vi "Display Error.vi"(6 "Show \"Ignore Error\" (T)":bool=TRUE, 10 "Error to Display":errorcluster, 11 "Title (\"\")":string) -> (2 "Ignore Error":bool, 3 "Exit?":bool)   [LabVIEW 2018]
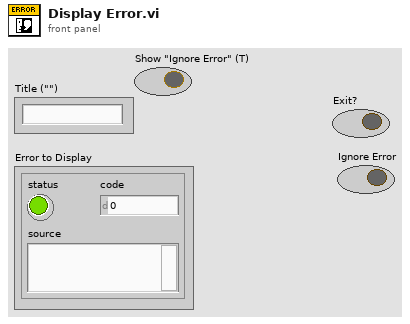
[diagram p1: front panel]
types:
  T1 = enum16{"Left Button", "Center Button", "Right Button", "Window Close"}
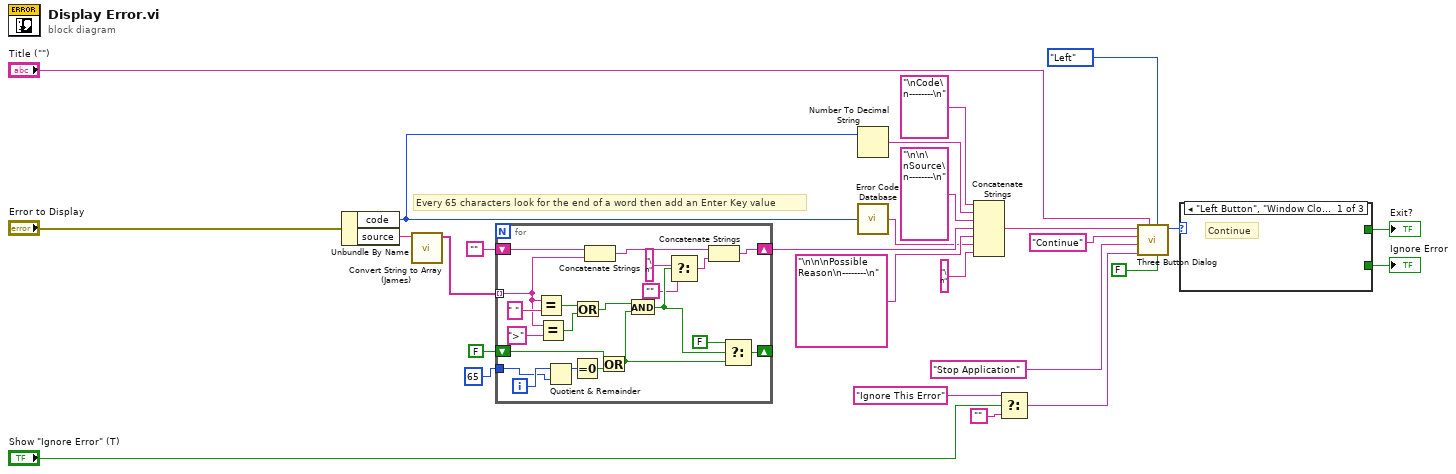
[diagram p0: block diagram]
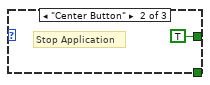
[diagram p2: hidden frame]
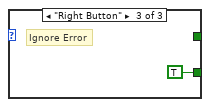
[diagram p3: hidden frame]
diagram:
  # "Every 65 characters look for the end of a word then add an Enter Key value"
  n1 = Unbundle By Name("Error to Display") -> ("code"=w17:i32, "source"=w20:string)
  n2 = call "Convert String to Array (James).vi"("String in"=w20) -> ("Array out"=w24:string[])  [unwired: 9 in, 1 out]
  n3 = for {
    tunnel: w24 -> [w42] mode=indexing
    shift-right: [w39] -> w19
    shift-left: "" -> [w47]
    tunnel: 65 ("length") -> [w28]
    shift-right: [w37] -> _
    shift-left: FALSE -> [w33]
    i -> [w29]
    n4 = Equal?(x=w42, y=" ") -> (x = y?=w43:bool)
    n5 = Equal?(x=w42, y=">") -> (x = y?=w40:bool)
    n6 = Quotient & Remainder(x=w29, y=w28) -> (x-y*floor(x/y)=w46:i32)  [unwired: 1 out]
    n7 = Equal To 0?(x=w46) -> (x = 0?=w45:bool)
    n8 = Or(x=w43, y=w40) -> (x .or. y?=w34:bool)
    n9 = Concatenate Strings(w47, w42) -> (w48:string)
    n10 = Or(x=w33, y=w45) -> (x .or. y?=w32:bool)
    n11 = And(x=w34, y=w32) -> (x .and. y?=w38:bool)
    n12 = Select(t="\n", s=w38, f="") -> (s? t:f=w35:string)
    n13 = Concatenate Strings(w48, w35) -> (w39:string)
    n14 = Select(t=FALSE, s=w38, f=w32) -> (s? t:f=w37:bool)
  }
  n15 = Number To Decimal String(number=w17) -> (decimal integer string=w27:string)  [unwired: 1 in]
  n16 = call <vilib>:"Error Code Database.vi"("Error Code"=w17) -> ("Error Text"=w16:string)
  n17 = Concatenate Strings("\nCode\n--------\n", w27, "\n\n\nSource\n--------\n", w19, "\n\n\nPossible Reason\n--------\n" ("string"), w16, "\n" ("string")) -> (w10:string)
  n18 = Select(t="Ignore This Error" ("Right Button Text (\"Cancel\")"), s="Show \"Ignore Error\" (T)", f="") -> (s? t:f=w1:string)
  n19 = call <vilib>:"Three Button Dialog.vi"("Allow user to close window? (TRUE)"=FALSE, "Justify Message (Left)"=enum16{"Left", "Center", "Right"}."Left" ("Justify Message (Center)"), "Window Title (\"\")"="Title (\"\")", "Right Button Text (\"Cancel\")"=w1, "Center Button Text (\"No\")"="Stop Application" ("T button name (\"OK\")"), "Left Button Text (\"Yes\")"="Continue" ("F button name (\"Cancel\")"), "message"=w10) -> ("Which Button?"=w7:T1)  [unwired: 4 in]
  n20 = case shown="\"Left Button\", \"Window Close\", Default" w7 {
    tunnel: [_ TRUE _] -> w6
    tunnel: [_ _ TRUE] -> w5
    frame "Left Button", "Window Close", Default {
      # "Continue"
    }
    frame "Center Button" {
      # "Stop Application"
    }
    frame "Right Button" {
      # "Ignore Error"
    }
  }
  "Exit?" <- w6
  "Ignore Error" <- w5
